vi "Prepare RProp.vi"(11 "Neural Network In":T1) -> (2 "Teach Coef Buffer":T2[](array[typedef]), 3 "Gradient Buffer":T2[](array[typedef]))   [LabVIEW 2011, in "Super Simple Neural Network.lvlib"]
uses:
  Super Simple Neural Network.lvlib
  Types/2D Array.ctl
  Types/Neural Network.ctl
  Types/Scaling Info.ctl
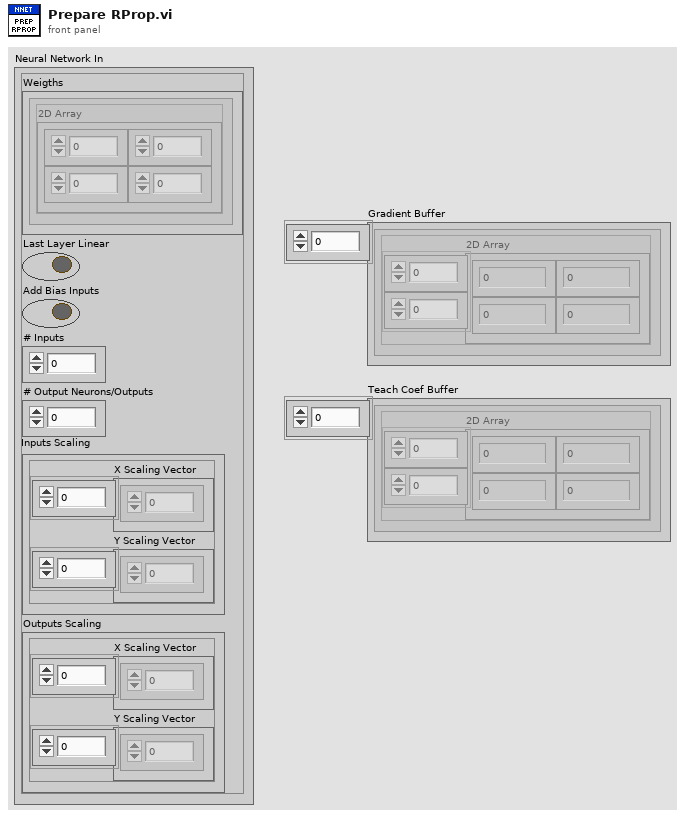
[diagram p1: front panel]
types:
  T1 = typedef "Super Simple Neural Network.lvlib/Neural Network.ctl" = cluster{"Weigths":T2[], "Last Layer Linear":bool, "Add Bias Inputs":bool, "# Inputs":u32, "# Output Neurons/Outputs":u32, "Inputs Scaling":T3, "Outputs Scaling":T3}
  T2 = typedef "Super Simple Neural Network.lvlib/2D Array.ctl" = cluster{"2D Array":dbl[][]}
  T3 = typedef "Super Simple Neural Network.lvlib/Scaling Info.ctl" = cluster{"X Scaling Vector":dbl[], "Y Scaling Vector":dbl[]}
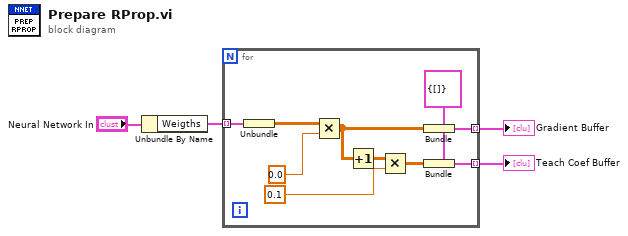
[diagram p0: block diagram]
diagram:
  n1 = Unbundle By Name("Neural Network In") -> ("Weigths"=w1:T2[])
  n2 = for {
    tunnel: w1 -> [w14] mode=indexing
    tunnel: [w11] -> w3 mode=indexing
    tunnel: [w5] -> w4 mode=indexing
    w10 = T2 {"2D Array"=[]}
    n3 = Unbundle(w14) -> ("2D Array"=w12:dbl[][])
    n4 = Multiply(x=w12, y=0.0) -> (x*y=w8:dbl[][])
    n5 = Increment(x=w8) -> (x+1=w9:dbl[][])
    n6 = Multiply(x=w9, y=0.1) -> (x*y=w6:dbl[][])
    n7 = Bundle(cluster=w10, "2D Array"=w8) -> (w11:T2)
    n8 = Bundle(cluster=w10, "2D Array"=w6) -> (w5:T2)
  }
  "Teach Coef Buffer" <- w4
  "Gradient Buffer" <- w3
